vi "Read HttpHeaders.vi"(8 "error in (no error)":errorcluster, 11 "HttpRequestMessage in":refnum<class "HttpRequestMessage.lvclass">) -> (0 "error out":errorcluster, 2 "HttpHeaders":refnum<class "HttpHeaders_Request.lvclass">, 3 "HttpRequestMessage out":refnum<class "HttpRequestMessage.lvclass">)   [LabVIEW 2018, in "HttpClient_NET.lvlib" / "HttpRequestMessage.lvclass"]
uses:
  HttpRequestMessage.lvclass
  HttpHeaders_Request/HttpHeaders_Request.lvclass
  C:/Viviota/Projects/R&D/LabVIEW_HTTP_REST_NET/HTTPHeaders_NET/HttpHeaders_NET.lvclass
  HttpRequestMessage.lvclass/HttpRequestMessage.ctl
  System.Net.Http
  HTTPHeaders_NET/HttpHeaders_NET.lvclass
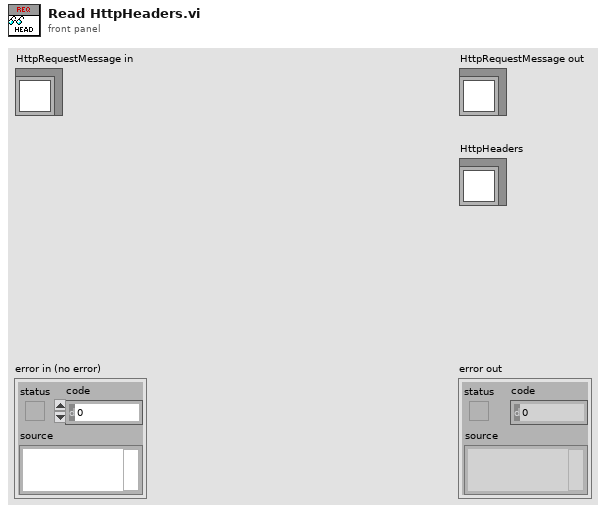
[diagram p1: front panel]
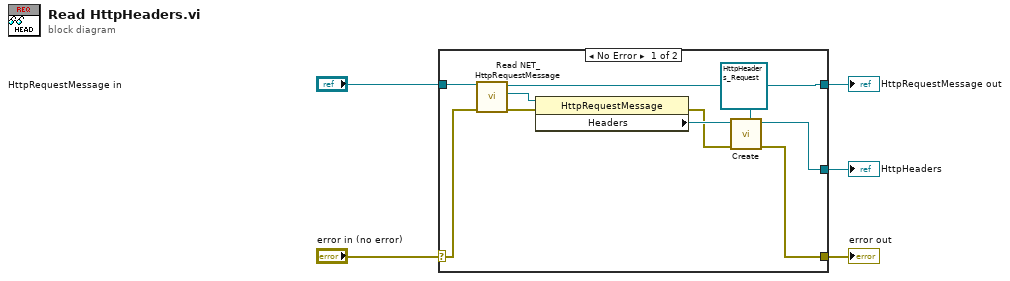
[diagram p0: block diagram]
diagram:
  n1 = case shown="No Error" "error in (no error)" {
    selector: "error in (no error)" -> [w8 w16]
    tunnel: [w6 w16] -> w4
    tunnel: [w10 w17] -> w2
    tunnel: "HttpRequestMessage in" -> [w15 w17]
    tunnel: [w9 _] -> w1
    frame No Error {
      n2 = call "Read NET_HttpRequestMessage.vi"("error in (no error)"=w8, "HttpRequestMessage in"=w15) -> ("error out"=w14:errorcluster, "NET_HttpRequestMessage"=w13:refnum<k24>, "HttpRequestMessage out"=w10:refnum<class "HttpRequestMessage.lvclass">)  [unwired: 7 in]
      n3 = property class="HttpRequestMessage"(reference=w13, error in=w14) -> (error out=w7:errorcluster, "Headers"=w12:refnum<k24>)  [unwired: 1 out]
      n4 = call "Create.vi"("HTTPHeaders_NET in"=refnum<class "HttpHeaders_Request.lvclass"> refnum ("LabVIEWHTTPClient_NET.lvlib:HttpHeaders_Request.lvclass"), "error in (no error)"=w7, "NET_HttpHeaders"=w12) -> ("error out"=w6:errorcluster, "HTTPHeaders_NET out"=w9:refnum<class "HttpHeaders_Request.lvclass">)  [unwired: 7 in]
    }
    frame Error {
    }
  }
  "error out" <- w4
  "HttpRequestMessage out" <- w2
  "HttpHeaders" <- w1
